vi "Identify Blocked Columns.vi"(11 "Nearest Point per Column":dbl[](array[numeric])=[inf, inf, inf, inf, inf, inf, inf, inf, 1479.5118855614214, 1478.374339038341, 1483.0270714842827, 1481.994560024077, 1482.1803311567019, 1479.0770828687473, inf, inf, inf, inf, inf, inf, inf, inf, inf, inf, inf, inf, inf, inf, inf, inf, inf, inf, inf, 1481.2550739106473, 1493.9549836722085, 1481.746288490731, 1481.6801013756658, 1481.4393767634901, 1477.2121936542683, 1483.476673653026, 1490.0109678222693, 1491.0446880125241, 1493.9871246951943, 1493.0530117205722, 1494.6270330949292, 1488.0944353045472, 1489.7344287216215, inf, inf, inf]) -> (0 "Goal Y":dbl=1477.2121936542683, 3 "Blocked Columns":bool[](array[boolean]))   [LabVIEW 2017]
panel:
  in  "Lookahead Threshold":dbl=150.0 format="%#_13g"
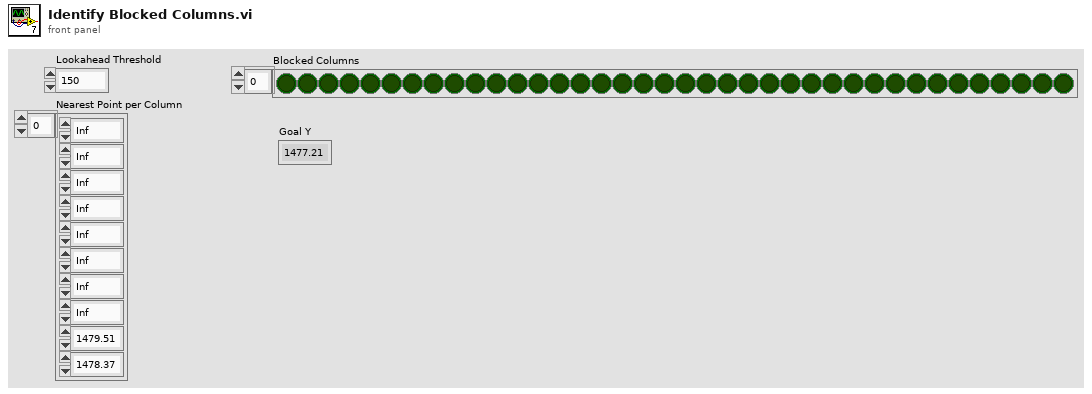
[diagram p1: front panel]
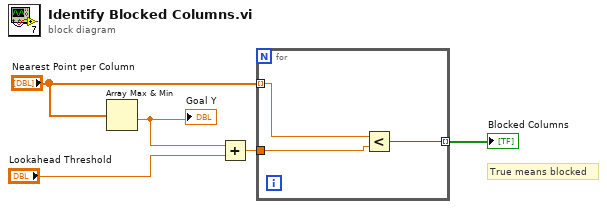
[diagram p0: block diagram]
diagram:
  # "True means blocked"
  n1 = Array Max & Min(array="Nearest Point per Column") -> (min value=w5:dbl)  [unwired: 3 out]
  "Goal Y" <- w5
  n2 = Add(x=w5, y="Lookahead Threshold") -> (x+y=w3:dbl)
  n3 = for {
    tunnel: w3 -> [w8]
    tunnel: "Nearest Point per Column" -> [w7] mode=indexing
    tunnel: [w6] -> w1 mode=indexing
    n4 = Less?(x=w7, y=w8) -> (x < y?=w6:bool)
  }
  "Blocked Columns" <- w1
